vi "Calculate BIN DISTANCE XYZ Keep Best Ver01.vi"(9 "KEEP X Best Points\nfor EACH BIN":i32=1, 10 "Data (X,Y,Z)":dbl[][](array[numeric]), 11 "BIN (X,Y,Z)":dbl[][](array[numeric])) -> (3 "Duplicate Points ELIMINATED":dbl[][](array[numeric]))   [LabVIEW 2017]
panel:
  in  "Tab Control":enum32{"Page 1", "Page 2"}(tab)
  out "BEST Points in each BIN\n(Distance, BIN#, POINT#)":dbl[][](array[numeric])
  out "ALL DISTANCE, BIN#, POINT#":dbl[][](array[numeric])
  out "BEST Points SORTED BY POINT#":dbl[][](array[numeric])
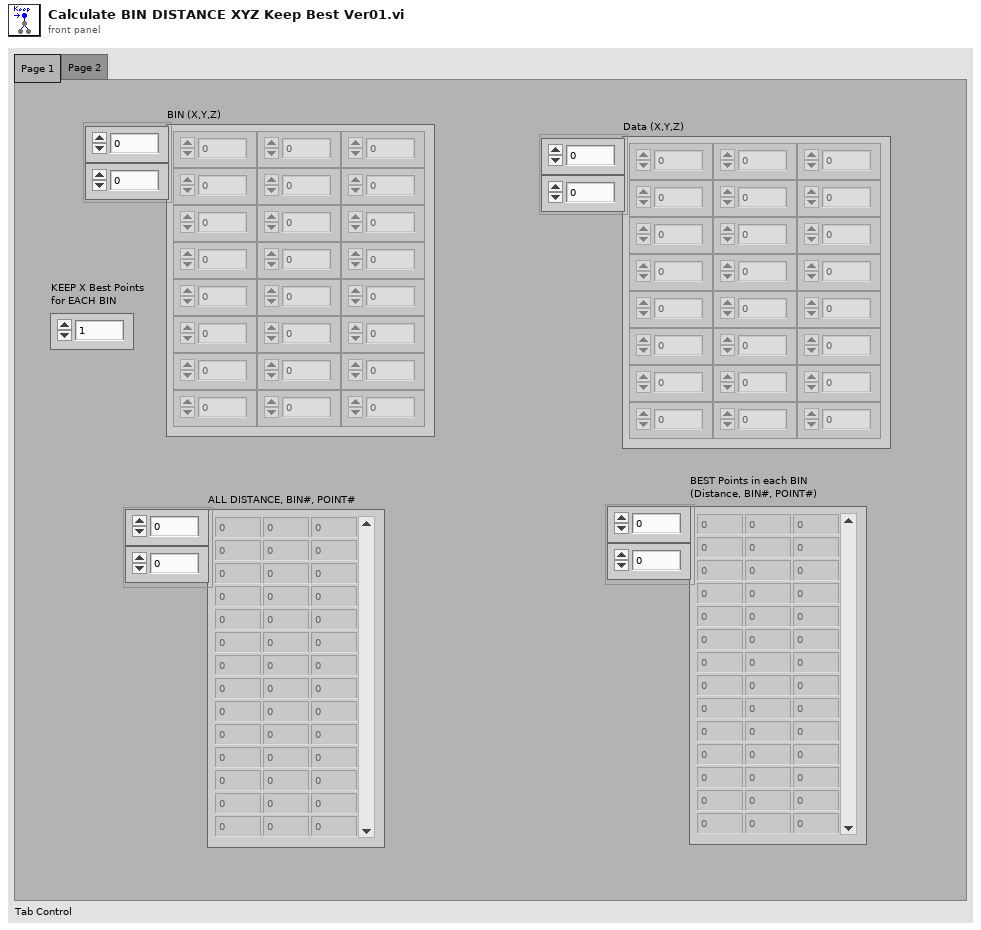
[diagram p1: front panel]
types:
  T1 = cluster{"[0]":dbl, "[1]":dbl, "[2]":dbl, "[3]":dbl, "[4]":dbl, "[5]":dbl, "[6]":dbl, "[7]":dbl, "[8]":dbl}
  T2 = cluster{"[0]":dbl, "[1]":dbl, "[2]":dbl, "[3]":dbl, "[4]":dbl, "[5]":dbl, "[6]":dbl, "[7]":dbl, "[8]":dbl}[]
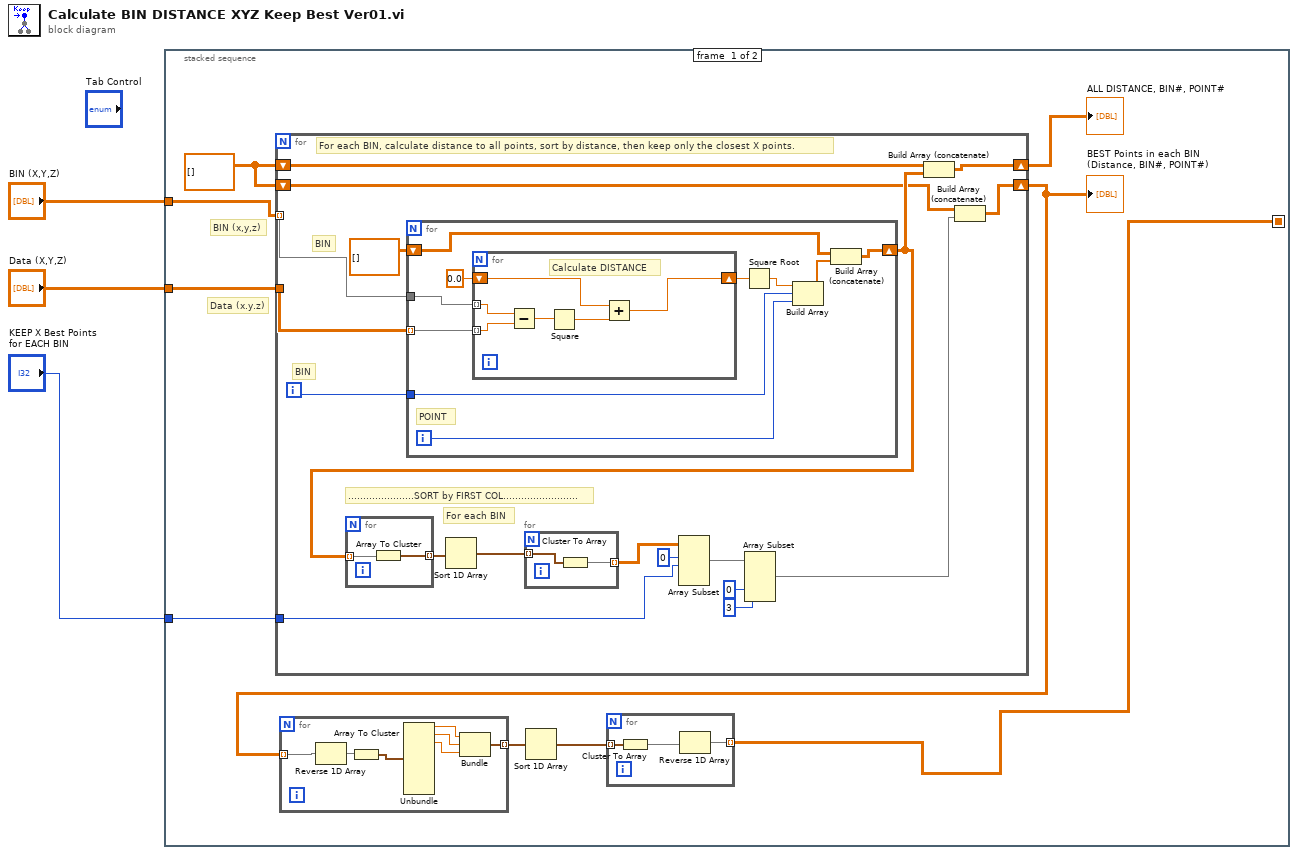
[diagram p0: block diagram]
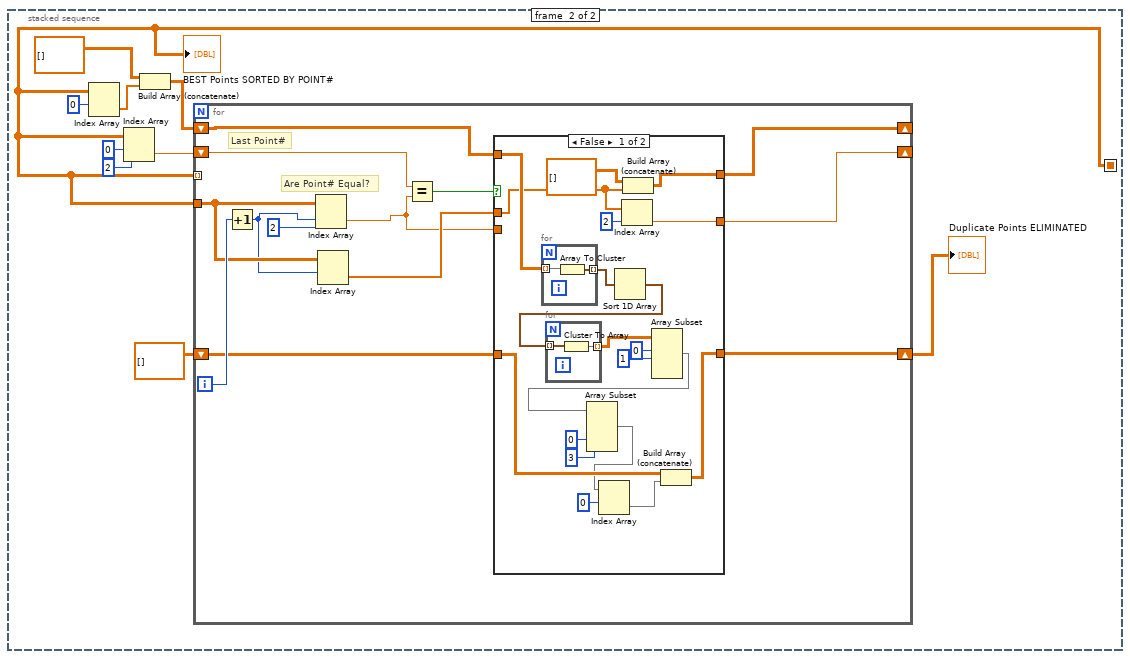
[diagram p2: hidden frame]
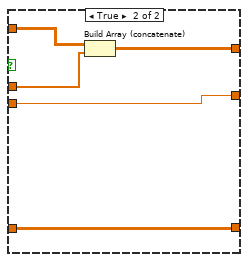
[diagram p3: hidden frame]
diagram:
  n1 = stacked-sequence {
    seq-local: [w5 _] -> [_ w67]
    tunnel: "BIN (X,Y,Z)" -> [w11 _]
    tunnel: "Data (X,Y,Z)" -> [w10 _]
    tunnel: "KEEP X Best Points\nfor EACH BIN" -> [w8 _]
    frame #0 {
      w9 = dbl[][] []
      # "Data (x.y.z)"
      # "BIN (x,y,z)"
      n2 = for {
        tunnel: w11 -> [w39] mode=indexing
        tunnel: w10 -> [w40]
        shift-right: [w37] -> w12
        shift-left: w9 -> [w36]
        shift-right: [w29] -> w4
        shift-left: w9 -> [w30]
        tunnel: w8 -> [w27]
        i -> [w35]
        # "For each BIN"
        # "......................SORT by FIRST COL........................."
        # "BIN"
        # "BIN"
        # "For each BIN, calculate distance to all points, sort by distance, then keep only the closest X points."
        n3 = for {
          tunnel: w40 -> [w53] mode=indexing
          tunnel: w39 -> [w54]
          shift-right: [w48] -> w31
          shift-left: dbl[][] [] -> [w47]
          tunnel: w35 -> [w46]
          i -> [w45]
          # "POINT"
          n4 = for {
            tunnel: w54 -> [w60] mode=indexing
            tunnel: w53 -> [w59] mode=indexing
            shift-right: [w56] -> w51
            shift-left: 0.0 -> [w55]
            # "Calculate DISTANCE"
            n5 = Subtract(x=w60, y=w59) -> (x-y=w58:dbl)
            n6 = Square(x=w58) -> (x^2=w57:dbl)
            n7 = Add(x=w55, y=w57) -> (x+y=w56:dbl)
          }
          n8 = Square Root(x=w51) -> (sqrt(x)=w50:dbl)
          n9 = Build Array(w50, w46, w45) -> (w49:dbl[])
          n10 = Build Array (concatenate)(w47, w49) -> (w48:dbl[][])
        }
        n11 = for {
          tunnel: w31 -> [w44] mode=indexing
          tunnel: [w43] -> w33 mode=indexing
          n12 = Array To Cluster(array=w44) -> (cluster=w43:T1)
        }
        n13 = Sort 1D Array(array=w33) -> (sorted array=w34:T2)
        n14 = for {
          tunnel: w34 -> [w42] mode=indexing
          tunnel: [w41] -> w32 mode=indexing
          n15 = Cluster To Array(cluster=w42) -> (array=w41:dbl[])
        }
        n16 = Array Subset(array=w32, index (row)=0 ("index"), length (row)=w27) -> (w26:dbl[][])  [unwired: 2 in]
        n17 = Array Subset "Array Subset"(array=w26, index (col)=0 ("index"), length (col)=3 ("length")) -> (w23:dbl[][])  [unwired: 2 in]
        n18 = Build Array (concatenate)(w36, w31) -> (w37:dbl[][])
        n19 = Build Array (concatenate)(w30, w23) -> (w29:dbl[][])
      }
      "ALL DISTANCE, BIN#, POINT#" <- w12
      "BEST Points in each BIN\n(Distance, BIN#, POINT#)" <- w4
      n20 = for {
        tunnel: w4 -> [w22] mode=indexing
        tunnel: [w20] -> w7 mode=indexing
        n21 = Reverse 1D Array(array=w22) -> (reversed array=w21:dbl[])
        n22 = Array To Cluster(array=w21) -> (cluster=w19:T1)
        n23 = Unbundle(w19) -> ("[0]"=w18:dbl, "[1]"=w17:dbl, "[2]"=w16:dbl)  [unwired: 6 out]
        n24 = Bundle("[0]"=w18, "[1]"=w17, "[2]"=w16) -> (w20:cluster{"[0]":dbl, "[1]":dbl, "[2]":dbl})  [unwired: 1 in]
      }
      n25 = Sort 1D Array(array=w7) -> (sorted array=w6:cluster{"[0]":dbl, "[1]":dbl, "[2]":dbl}[])
      n26 = for {
        tunnel: w6 -> [w15] mode=indexing
        tunnel: [w13] -> w5 mode=indexing
        n27 = Cluster To Array(cluster=w15) -> (array=w14:dbl[])
        n28 = Reverse 1D Array(array=w14) -> (reversed array=w13:dbl[])
      }
    }
    frame #1 {
      n29 = Index Array(array=w67, index (row)=0) -> (element=w64:dbl[])  [unwired: 1 in]
      n30 = Index Array(array=w67, index (row)=0, index (col)=2 ("disabled index (col)")) -> (element=w68:dbl)
      n31 = Build Array (concatenate)(dbl[][] [], w64) -> (w63:dbl[][])
      n32 = for {
        tunnel: w67 -> [_] mode=indexing
        tunnel: w67 -> [w78]
        shift-right: [w72] -> _
        shift-left: w68 -> [w81]
        shift-right: [w79] -> _
        shift-left: w63 -> [w75]
        shift-right: [w74] -> w61
        shift-left: dbl[][] [] -> [w73]
        i -> [w82]
        # "Last Point#"
        # "Are Point# Equal?"
        n33 = Increment(x=w82) -> (x+1=w77:i32)
        n34 = Index Array(array=w78, index (row)=w77, index (col)=2) -> (element=w71:dbl)
        n35 = Index Array(array=w78, index (row)=w77) -> (element=w76:dbl[])  [unwired: 1 in]
        n36 = Equal?(x=w81, y=w71) -> (x = y?=w80:bool)
        n37 = case shown="False" w80 {
          tunnel: [w101 w111] -> w79
          tunnel: w76 -> [w94 w109]
          tunnel: w75 -> [w100 w110]
          tunnel: [w84 w108] -> w74
          tunnel: w73 -> [w88 w108]
          tunnel: [w92 w107] -> w72
          tunnel: w71 -> [_ w107]
          frame False {
            n38 = for {
              tunnel: w100 -> [w106] mode=indexing
              tunnel: [w105] -> w99 mode=indexing
              n39 = Array To Cluster(array=w106) -> (cluster=w105:T1)
            }
            n40 = Sort 1D Array(array=w99) -> (sorted array=w98:T2)
            n41 = for {
              tunnel: w98 -> [w104] mode=indexing
              tunnel: [w103] -> w96 mode=indexing
              n42 = Cluster To Array(cluster=w104) -> (array=w103:dbl[])
            }
            n43 = Index Array(array=w94, index=2) -> (element=w92:dbl)
            n44 = Build Array (concatenate)(dbl[][] [], w94) -> (w101:dbl[][])
            n45 = Array Subset(array=w96, index (row)=0 ("index"), length (row)=1 ("length")) -> (w89:dbl[][])  [unwired: 2 in]
            n46 = Array Subset "Array Subset"(array=w89, index (col)=0 ("index"), length (col)=3 ("length")) -> (w87:dbl[][])  [unwired: 2 in]
            n47 = Index Array(array=w87, index (row)=0) -> (element=w85:dbl[])  [unwired: 1 in]
            n48 = Build Array (concatenate)(w88, w85) -> (w84:dbl[][])
          }
          frame True {
            n49 = Build Array (concatenate)(w110, w109) -> (w111:dbl[][])
          }
        }
      }
      "Duplicate Points ELIMINATED" <- w61
      "BEST Points SORTED BY POINT#" <- w67
    }
  }
